vi "Create Instrument SMO.vi"(8 "error in (no error)":errorcluster, 9 "Debug Mode? [F]":bool, 10 "Configuration Window? [T]":bool=TRUE, 11 "Instrument in":refnum<class "Instrument.lvclass">) -> (0 "error out":errorcluster, 3 "Instrument out":refnum<class "Instrument.lvclass">)   [LabVIEW 2019, in "Instrument.lvlib" / "Instrument.lvclass"]
doc: "Create a new instance of your Instrument. A little bt of configuration happens before calling \"Create SMO.vi\""
uses:
  Instrument.lvclass
  C:/Program Files/National Instruments/LabVIEW 2019/vi.lib/JKI/JKI SMO/SMO/SMO.lvclass
  <vilib>/JKI/JKI SMO/SMO/SMO.lvclass
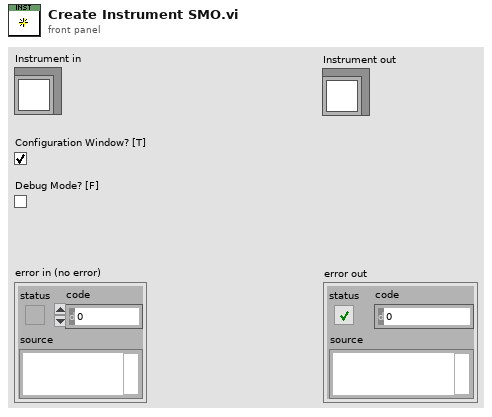
[diagram p1: front panel]
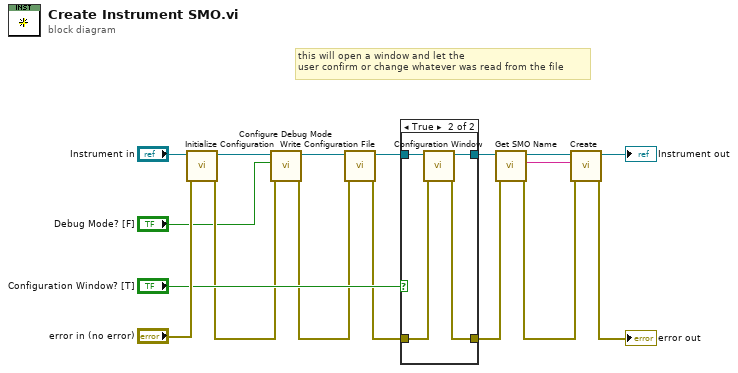
[diagram p0: block diagram]
diagram:
  # "this will open a window and let the\nuser confirm or change whatever was read from the file"
  n1 = call "Initialize Configuration.vi"("error in (no error)"="error in (no error)", "Instrument in"="Instrument in") -> ("error out"=w5:errorcluster, "Instrument out"=w2:refnum<class "Instrument.lvclass">)  [unwired: 8 in]
  n2 = call "Configure Debug Mode.vi"("error in (no error)"=w5, "Debug Mode? [F]"="Debug Mode? [F]", "Instrument in"=w2) -> ("error out"=w4:errorcluster, "Instrument out"=w3:refnum<class "Instrument.lvclass">)  [unwired: 7 in]
  n3 = call-dynamic "Write Configuration File.vi"("error in (no error)"=w4, "Instrument in"=w3) -> ("error out"=w7:errorcluster, "Instrument out"=w6:refnum<class "Instrument.lvclass">)  [unwired: 8 in]
  n4 = case shown="True" "Configuration Window? [T]" {
    tunnel: [w18 w20] -> w11
    tunnel: [w19 w23] -> w12
    tunnel: w6 -> [w19 w22]
    tunnel: w7 -> [w18 w21]
    frame False {
    }
    frame True {
      n5 = call-dynamic "Configuration Window.vi"("error in (no error)"=w21, "Instrument"=w22) -> ("error out"=w20:errorcluster, "Instrument out"=w23:refnum<class "Instrument.lvclass">)  [unwired: 8 in]
    }
  }
  n6 = call-dynamic "Get SMO Name.vi"("error in (no error)"=w11, "Instrument in"=w12) -> ("error out"=w9:errorcluster, "SMO Name"=w8:string, "Instrument out"=w10:refnum<class "Instrument.lvclass">)  [unwired: 7 in]
  n7 = call <vilib>:"Create.vi"("error in (no error)"=w9, "Subsystem Name (optional)"=w8, "SMO"=w10) -> ("error out"=→"error out":errorcluster, "SMO out"=→"Instrument out":refnum<class "Instrument.lvclass">)  [unwired: 6 in, 1 out]
